vi "compare.obs.vi"(10 "expected.OrderBooks.out":T2[](array[typedef]) {"Ask (Sell)"."OrderId" format="%.0x"; "Bid (Buy)"."OrderId" format="%.0x"}, 11 "actual.OrderBooks.out":T2[](array[typedef]) {"Ask (Sell)"."OrderId" format="%.0x"; "Bid (Buy)"."OrderId" format="%.0x"}) -> (2 "Results.detailed":T1(array[cluster]), 3 "Passed":bool)   [LabVIEW 2020]
uses:
  types/val.pretty.orderbook.ctl
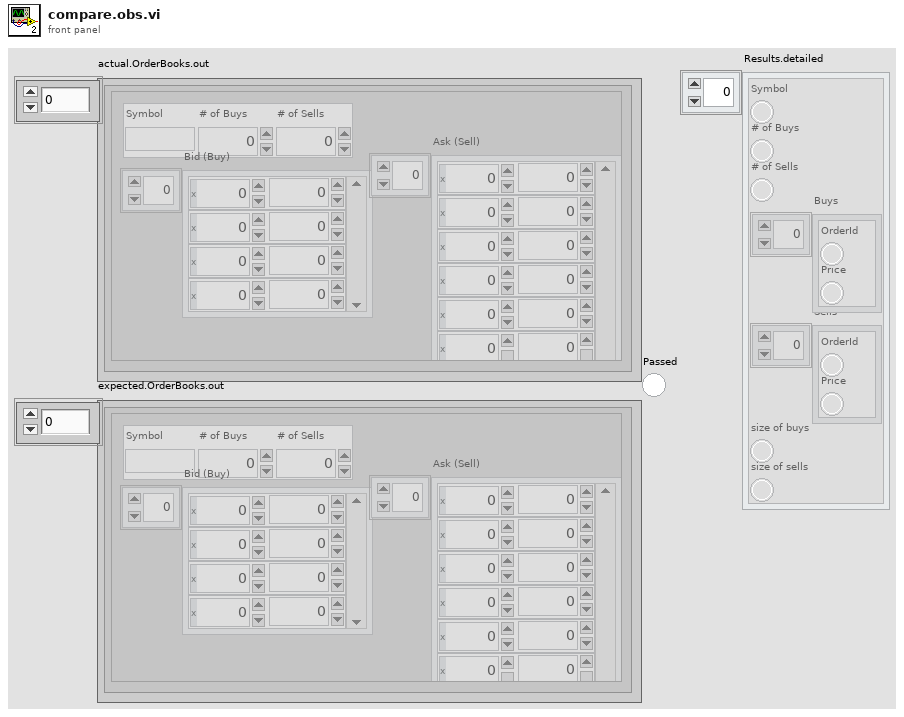
[diagram p1: front panel]
types:
  T1 = cluster{"Symbol":bool, "# of Buys":bool, "# of Sells":bool, "Buys":cluster{"OrderId":bool, "Price":bool}[], "Sells":cluster{"OrderId":bool, "Price":bool}[], "size of buys":bool, "size of sells":bool}[]
  T2 = typedef "val.pretty.orderbook.ctl" = cluster{"metadata":cluster{"Symbol":string, "# of Buys":u64, "# of Sells":u64}, "Bid (Buy)":cluster{"OrderId":u64, "Price":dbl}[], "Ask (Sell)":cluster{"OrderId":u64, "Price":dbl}[]}
  T3 = cluster{"Symbol":bool, "# of Buys":bool, "# of Sells":bool, "Buys":cluster{"OrderId":bool, "Price":bool}[], "Sells":cluster{"OrderId":bool, "Price":bool}[], "size of buys":bool, "size of sells":bool}
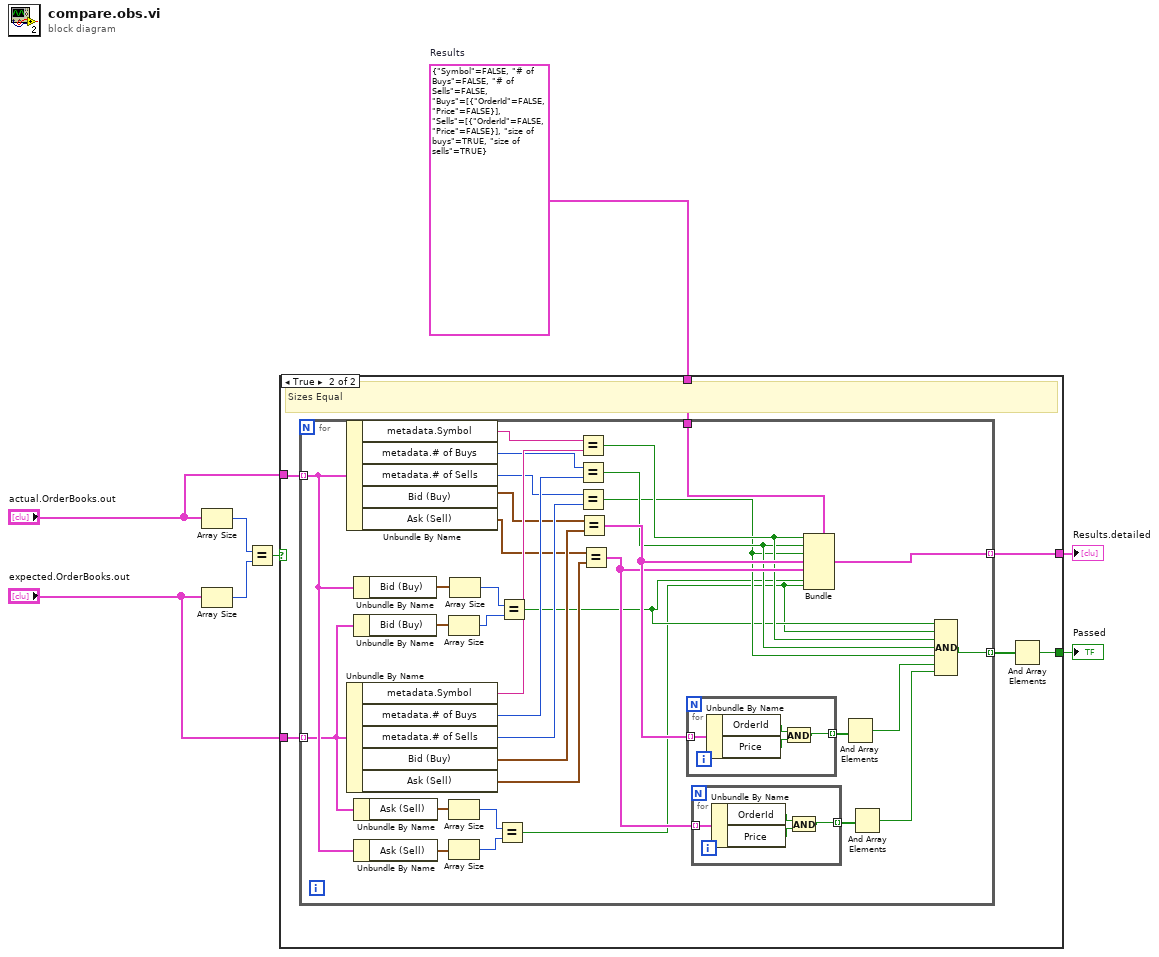
[diagram p0: block diagram]
diagram:
  w3 = T3 {"Symbol"=FALSE, "# of Buys"=FALSE, "# of Sells"=FALSE, "Buys"=[{"OrderId"=FALSE, "Price"=FALSE}], "Sells"=[{"OrderId"=FALSE, "Price"=FALSE}], "size of buys"=TRUE, "size of sells"=TRUE}  # Results
  n1 = Array Size(array="actual.OrderBooks.out") -> (size(s)=w7:i32)
  n2 = Array Size(array="expected.OrderBooks.out") -> (size(s)=w8:i32)
  n3 = Equal?(x=w7, y=w8) -> (x = y?=w6:bool)
  n4 = case shown="True" w6 {
    tunnel: "actual.OrderBooks.out" -> [_ w14]
    tunnel: "expected.OrderBooks.out" -> [_ w13]
    tunnel: [_ w12] -> w1
    tunnel: w3 -> [_ w11]
    tunnel: [_ w9] -> w2
    frame False {
      # "Sizes not equal"
    }
    frame True {
      # "Sizes Equal"
      n5 = for {
        tunnel: w14 -> [w22] mode=indexing
        tunnel: w13 -> [w21] mode=indexing
        tunnel: [w38] -> w12 mode=indexing
        tunnel: w11 -> [w37]
        tunnel: [w27] -> w10 mode=indexing
        n6 = Unbundle By Name(w22) -> ("metadata.Symbol"=w48:string, "metadata.# of Buys"=w46:u64, "metadata.# of Sells"=w44:u64, "Bid (Buy)"=w42:cluster{"OrderId":u64, "Price":dbl}[], "Ask (Sell)"=w40:cluster{"OrderId":u64, "Price":dbl}[])
        n7 = Unbundle By Name(w21) -> ("metadata.Symbol"=w47:string, "metadata.# of Buys"=w45:u64, "metadata.# of Sells"=w43:u64, "Bid (Buy)"=w41:cluster{"OrderId":u64, "Price":dbl}[], "Ask (Sell)"=w39:cluster{"OrderId":u64, "Price":dbl}[])
        n8 = Unbundle By Name(w22) -> ("Bid (Buy)"=w26:cluster{"OrderId":u64, "Price":dbl}[])
        n9 = Unbundle By Name(w21) -> ("Bid (Buy)"=w25:cluster{"OrderId":u64, "Price":dbl}[])
        n10 = Unbundle By Name(w21) -> ("Ask (Sell)"=w20:cluster{"OrderId":u64, "Price":dbl}[])
        n11 = Unbundle By Name(w22) -> ("Ask (Sell)"=w19:cluster{"OrderId":u64, "Price":dbl}[])
        n12 = Array Size(array=w25) -> (size(s)=w24:i32)
        n13 = Array Size(array=w20) -> (size(s)=w18:i32)
        n14 = Array Size(array=w19) -> (size(s)=w17:i32)
        n15 = Array Size(array=w26) -> (size(s)=w23:i32)
        n16 = Equal?(x=w18, y=w17) -> (x = y?=w15:bool)
        n17 = Equal?(x=w23, y=w24) -> (x = y?=w16:bool)
        n18 = Equal?(x=w48, y=w47) -> (x = y?=w32:bool)
        n19 = Equal?(x=w46, y=w45) -> (x = y?=w31:bool)
        n20 = Equal?(x=w44, y=w43) -> (x = y?=w30:bool)
        n21 = Equal?(x=w42, y=w41) -> (x = y?=w36:cluster{"OrderId":bool, "Price":bool}[])
        n22 = Equal?(x=w40, y=w39) -> (x = y?=w34:cluster{"OrderId":bool, "Price":bool}[])
        n23 = for {
          tunnel: w36 -> [w56] mode=indexing
          tunnel: [w53] -> w35 mode=indexing
          n24 = Unbundle By Name(w56) -> ("OrderId"=w55:bool, "Price"=w54:bool)
          n25 = And(x=w55, y=w54) -> (x .and. y?=w53:bool)
        }
        n26 = for {
          tunnel: w34 -> [w52] mode=indexing
          tunnel: [w49] -> w33 mode=indexing
          n27 = Unbundle By Name(w52) -> ("OrderId"=w51:bool, "Price"=w50:bool)
          n28 = And(x=w51, y=w50) -> (x .and. y?=w49:bool)
        }
        n29 = Bundle(cluster=w37, "Symbol"=w32, "# of Buys"=w31, "# of Sells"=w30, "Buys"=w36, "Sells"=w34, "size of buys"=w16, "size of sells"=w15) -> (w38:T3)
        n30 = And Array Elements(Boolean array=w35) -> (logical AND=w29:bool)
        n31 = And Array Elements(Boolean array=w33) -> (logical AND=w28:bool)
        n32 = Compound Arithmetic op=AND(w16, w15, w32, w31, w30, w29, w28) -> (w27:bool)
      }
      n33 = And Array Elements(Boolean array=w10) -> (logical AND=w9:bool)
    }
  }
  "Passed" <- w2
  "Results.detailed" <- w1
